vi "PwF_ToF_GetDistance.vi"(0 "PwF ToF Ref":T1, 11 "error in (no error)":errorcluster) -> (4 "PwF ToF Ref":T1, 6 "Dist_mm":u16, 8 "RangingStatus":u8, 10 "MeasQuality":u8, 14 "SigRetRate":dbl, 15 "error out":errorcluster)   [LabVIEW 2018]
uses:
  ToF_TypeDef/PwF ToF Ref.ctl
  ToF_TypeDef/PwF ToF RangingMode.ctl
panel:
  out "DataAge_ms":u32
  out "Message ID Out":u32 format="%.0x"
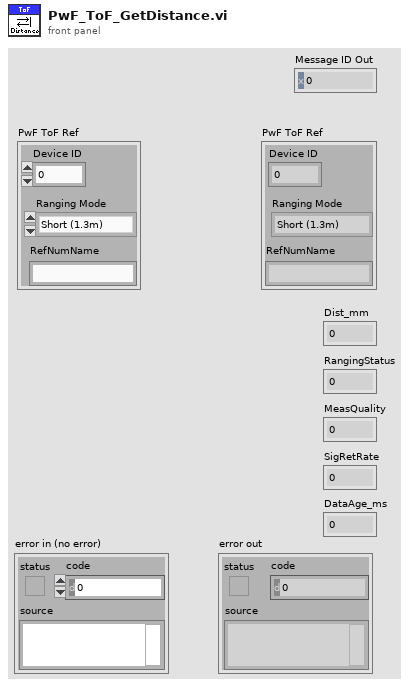
[diagram p1: front panel]
types:
  T1 = typedef "PwF ToF Ref.ctl" = cluster{"Device ID":u8, "Ranging Mode":T2, "RefNumName":string}
  T2 = typedef "PwF ToF RangingMode.ctl" = enum8{"Short (1.3m)", "Medium (2m)", "Long (4m)"}
  T3 = cluster{"Data[0]":u8, "Data[1]":u8, "Data[2]":u8, "Data[3]":u8, "Data[4]":u8, "Data[5]":u8, "Data[6]":u8, "Data[7]":u8, "Data[8]":u8}
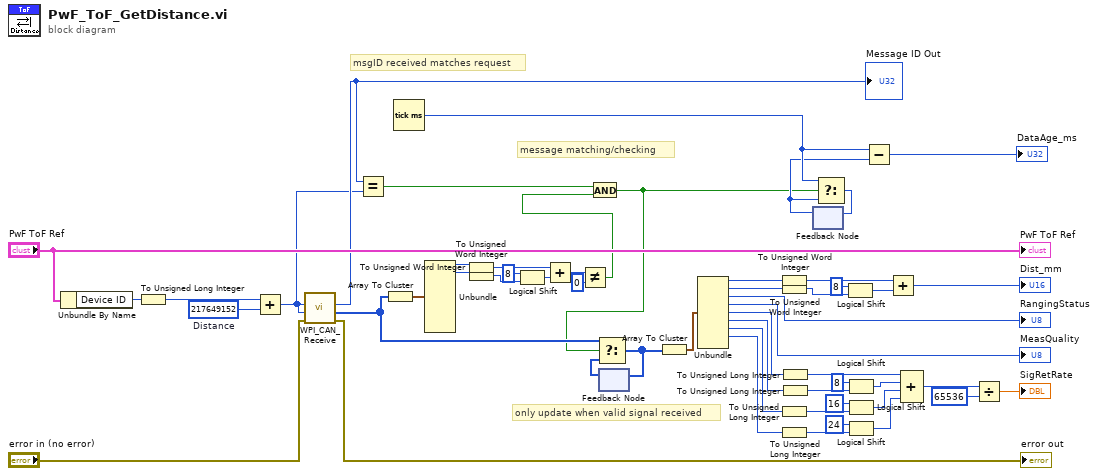
[diagram p0: block diagram]
diagram:
  w16 = u32 217649152  # Distance
  # "message matching/checking"
  # "only update when valid signal received"
  # "msgID received matches request"
  n1 = Unbundle By Name("PwF ToF Ref") -> ("Device ID"=w54:u8)
  n2 = To Unsigned Long Integer(number=w54) -> (unsigned 32bit integer=w23:u32)
  n3 = Add(x=w23, y=w16) -> (x+y=w1:u32)
  n4 = call <vilib>:"WPI_CAN_Receive.vi"("error in (no error)"="error in (no error)", "Message ID Mask"=w1, "Message ID"=w1) -> ("error out"=→"error out":errorcluster, "Data"=w14:u8[], "Message ID Out"=w22:u32)  [unwired: 6 in]
  "Message ID Out" <- w22
  n5 = Equal?(x=w22, y=w1) -> (x = y?=w4:bool)
  n6 = Array To Cluster(array=w14) -> (cluster=w13:T3)
  n7 = Tick Count (ms)() -> (millisecond timer value=w19:u32)
  n8 = Unbundle(w13) -> ("Data[0]"=w9:u8, "Data[1]"=w8:u8)  [unwired: 7 out]
  n9 = To Unsigned Word Integer(number=w9) -> (unsigned 16bit integer=w10:u16)
  n10 = To Unsigned Word Integer(number=w8) -> (unsigned 16bit integer=w7:u16)
  n11 = Logical Shift(y=i16 8, x=w7) -> (x << y=w11:u16)
  n12 = Add(x=w10, y=w11) -> (x+y=w6:u16)
  n13 = Not Equal?(x=w6, y=u16 0) -> (x != y?=w3:bool)
  n14 = And(x=w4, y=w3) -> (x .and. y?=w2:bool)
  n15 = feedback #1() -> (w21:u8[])  [unwired: 1 in]
  n16 = Select(t=w14, s=w2, f=w21) -> (s? t:f=w15:u8[])
  n17 = feedback-in #1(w15) -> ()
  n18 = Array To Cluster(array=w15) -> (cluster=w39:T3)
  n19 = Unbundle(w39) -> ("Data[0]"=w38:u8, "Data[1]"=w41:u8, "Data[2]"=→"RangingStatus":u8, "Data[3]"=→"MeasQuality":u8, "Data[4]"=w32:u8, "Data[5]"=w29:u8, "Data[6]"=w30:u8, "Data[7]"=w31:u8)  [unwired: 1 out]
  n20 = To Unsigned Word Integer(number=w38) -> (unsigned 16bit integer=w37:u16)
  n21 = To Unsigned Word Integer(number=w41) -> (unsigned 16bit integer=w40:u16)
  n22 = To Unsigned Long Integer(number=w30) -> (unsigned 32bit integer=w35:u32)
  n23 = To Unsigned Long Integer(number=w31) -> (unsigned 32bit integer=w36:u32)
  n24 = To Unsigned Long Integer(number=w32) -> (unsigned 32bit integer=w33:u32)
  n25 = To Unsigned Long Integer(number=w29) -> (unsigned 32bit integer=w34:u32)
  n26 = feedback #2() -> (w18:u32)  [unwired: 1 in]
  n27 = Select(t=w19, s=w2, f=w18) -> (s? t:f=w20:u32)
  n28 = feedback-in #2(w20) -> ()
  n29 = Logical Shift(y=i16 8, x=w40) -> (x << y=w43:u16)
  n30 = Logical Shift(y=i16 8, x=w34) -> (x << y=w49:u32)
  n31 = Logical Shift(y=i16 16, x=w35) -> (x << y=w48:u32)
  n32 = Logical Shift(y=i16 24, x=w36) -> (x << y=w47:u32)
  n33 = Subtract(x=w19, y=w18) -> (x-y=→"DataAge_ms":u32)
  n34 = Add(x=w37, y=w43) -> (x+y=→"Dist_mm":u16)
  n35 = Compound Arithmetic op=ADD(w33, w49, w48, w47) -> (w44:u32)
  n36 = Divide(x=w44, y=u32 65536) -> (x/y=→"SigRetRate":dbl)
  "PwF ToF Ref" <- "PwF ToF Ref"
